vi "Configure Sensitivity.vi"(8 "error in (no error)":errorcluster, 10 "Sensse mode":u16(ring) items=["NORMAL", "MID", "HIGH1", "HIGH2", "HIGH3"], 11 "VISA resource name":refnum<visa-resource-name>) -> (0 "error out":errorcluster, 3 "VISA resource name out":refnum<visa-resource-name>)   [LabVIEW 2021, in "Ceyear.lvlib"]
doc: "Configures the frequency range defining its start frequency and its stop frequency. If the start frequency is equal to the stop frequency, then the spectrum analyzer operates in the time-domain mode. Otherwise, the spectrum analyzer operates in frequency-domain mode."
uses:
  <instrlib>/Ceyear/Ceyear.lvlib
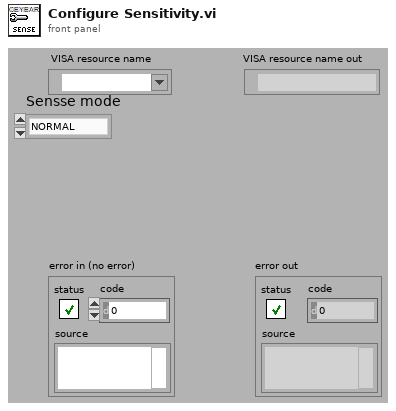
[diagram p1: front panel]
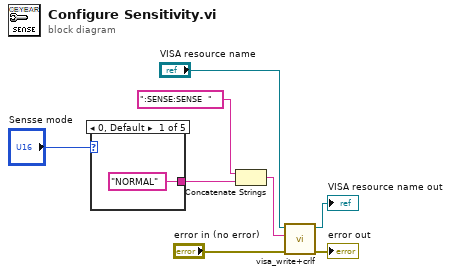
[diagram p0: block diagram]
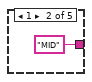
[diagram p2: hidden frame]
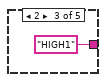
[diagram p3: hidden frame]
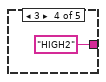
[diagram p4: hidden frame]
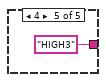
[diagram p5: hidden frame]
diagram:
  n1 = case shown="0, Default" "Sensse mode" {
    tunnel: ["NORMAL" "MID" "HIGH1" "HIGH2" "HIGH3"] -> w7
    frame 0, Default {
    }
    frame 1 {
    }
    frame 2 {
    }
    frame 3 {
    }
    frame 4 {
    }
  }
  n2 = Concatenate Strings(":SENSE:SENSE  ", w7) -> (w4:string)
  n3 = call <instrlib>:"visa_write+crlf.vi"("error in (no error)"="error in (no error)", "Strings (empty)"=w4, "VISA resource name"="VISA resource name") -> ("error out"=→"error out":errorcluster, "VISA resource name out"=→"VISA resource name out":refnum<visa-resource-name>)  [unwired: 7 in]
